vi "FGV Ausgaenge erzwingen.vi"(8 "Aktionen":T1) -> (0 "Aktionen":T1)   [LabVIEW 2020, in "cRIO Ueberwachung.lvlib"]
uses:
  cRIO Ueberwachung.lvlib
  FGV Ausgaenge erzwingen Aktionen.ctl
  Stoerungen/Stoerungen Messgeraet/Aktionen Kommunikation Stoerung.ctl
  Stoerungen/Stoerungen.lvlib
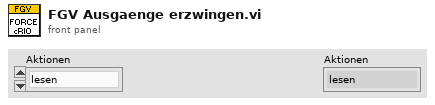
[diagram p1: front panel]
types:
  T1 = typedef "cRIO Ueberwachung.lvlib/FGV Ausgaenge erzwingen Aktionen.ctl" = enum16{"lesen", "starten", "erzwingen", "beenden"}
  T2 = typedef "Stoerungen.lvlib/Aktionen Kommunikation Stoerung.ctl" = enum16{"lesen", "init", "FT-IR Komm", "FT-IR Betriebsart", "FT-IR Hintergrund", "cRIO Komm", "PNS Komm", "Dichtheitstest", "Life Bit", "FTIR Komm AK", "PMA Komm", "FID Komm", "PMA Cal", "FID Ch4 Cal", "FID THC Cal", "Cal Timeout", "VFS 1 Komm", "VFS 2 Komm", "VFS 3 Komm", "VFS 4 Komm", "TRE 08 Komm", "CG-Test vorzeitig", "CG-Test Span 1", "CG-Test Span 2", "CG-Test Span 3", "CG-Test Messgas", "CG-Test löschen", "Test", "Amium AK", "AK Recept konfig", "AK Name konfig", "AK EKFG konfig"}
  T3 = typedef "Stoerungen.lvlib/Stoerungen Messgeraete.ctl" = cluster{"FT-IR Komm":bool, "FT-IR Betriebsart":bool, "FT-IR Hintergrundscan":bool, "Dichtheitstest":bool, "cRIO Komm":bool, "PNS Komm":bool, "Life Bit":bool, "FT-IR AK Komm":bool, "PMA Komm":bool, "FID Komm":bool, "PMA Cal":bool, "FID CH4 Cal":bool, "FID THC Cal":bool, "Cal Timeout":bool, "VFS 1 Komm":bool, "VFS 2 Komm":bool, "VFS 3 Komm":bool, "VFS 4 Komm":bool, "TRE 08 Komm":bool, "CG-Test":bool, "CG-Test 1":bool, "CG-Test 2":bool, "CG-Test 3":bool, "Messgas - Eingang":bool, "Amium AK Komm":bool, "AK Rezept nicht konfiguriert ":bool, "AK Name nicht konfiguriert":bool, "AK EKFG nicht konfiguriert":bool}
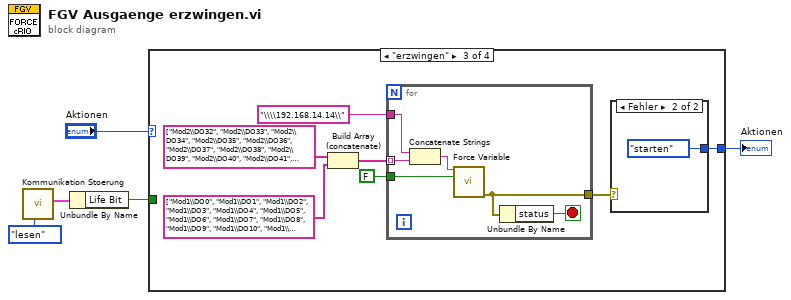
[diagram p0: block diagram]
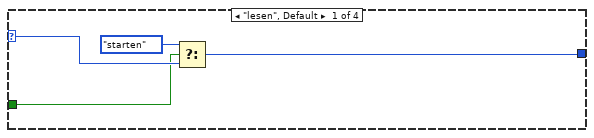
[diagram p2: hidden frame]
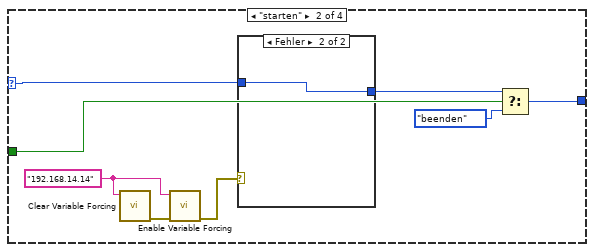
[diagram p3: hidden frame]
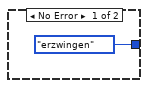
[diagram p4: hidden frame]
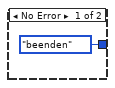
[diagram p5: hidden frame]
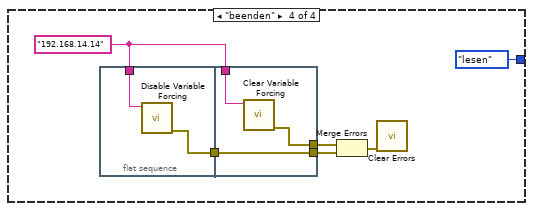
[diagram p6: hidden frame]
diagram:
  n1 = call "Kommunikation Stoerung.vi"("Aktionen"=Aktionen_Kommunikation_Stoerung."lesen") -> ("Störung Messgerät"=w3:T3)  [unwired: 10 in]
  n2 = Unbundle By Name(w3) -> ("Life Bit"=w1:bool)
  n3 = case shown="\"erzwingen\"" "Aktionen" {
    selector: "Aktionen" -> [w9 w12 _ _]
    tunnel: [w7 w10 w24 FGV_Ausgaenge_erzwingen_Aktionen."lesen" ("f")] -> w4
    tunnel: w1 -> [w6 w14 _ _]
    frame "lesen", Default {
      n4 = Select(t=FGV_Ausgaenge_erzwingen_Aktionen."starten", s=w6, f=w9) -> (s? t:f=w7:T1)
    }
    frame "starten" {
      w15 = "192.168.14.14"
      n5 = call <vilib>:"Clear Variable Forcing.vi"("target address (localhost)"=w15) -> ("error out"=w17:errorcluster)  [unwired: 1 in, 7 out]
      n6 = call <vilib>:"Enable Variable Forcing.vi"("error in (no error)"=w17, "target address (localhost)"=w15) -> ("error out"=w16:errorcluster)  [unwired: 7 out]
      n7 = case shown="Fehler" w16 {
        tunnel: [FGV_Ausgaenge_erzwingen_Aktionen."erzwingen" ("Aktionen") w19] -> w11
        tunnel: w12 -> [_ w19]
        frame No Error {
        }
        frame Error {
        }
      }
      n8 = Select(t=w11, s=w14, f=FGV_Ausgaenge_erzwingen_Aktionen."beenden") -> (s? t:f=w10:T1)
    }
    frame "erzwingen" {
      n9 = Build Array (concatenate)(string[] ["Mod2\\DO32", "Mod2\\DO33", "Mod2\\DO34", "Mod2\\DO35", "Mod2\\DO36", "Mod2\\DO37", "Mod2\\DO38", "Mod2\\DO39", "Mod2\\DO40", "Mod2\\DO41", "Mod2\\DO42", "Mod2\\DO43", "Mod2\\DO44", "Mod2\\DO45", "Mod2\\DO46", "Mod2\\DO47", "Mod3\\DO48", "Mod3\\DO49", "Mod3\\DO50", "Mod3\\DO51", "Mod3\\DO52", "Mod3\\DO53", "Mod3\\DO54", "Mod3\\DO55", "Mod3\\DO56", "Mod3\\DO57", "Mod3\\DO58", "Mod3\\DO59", "Mod3\\DO60", "Mod3\\DO61", "Mod3\\DO62", "Mod3\\DO63"], string[] ["Mod1\\DO0", "Mod1\\DO1", "Mod1\\DO2", "Mod1\\DO3", "Mod1\\DO4", "Mod1\\DO5", "Mod1\\DO6", "Mod1\\DO7", "Mod1\\DO8", "Mod1\\DO9", "Mod1\\DO10", "Mod1\\DO11", "Mod1\\DO12", "Mod1\\DO13", "Mod1\\DO14", "Mod1\\DO15", "Mod1\\DO16", "Mod1\\DO17", "Mod1\\DO18", "Mod1\\DO19", "Mod1\\DO20", "Mod1\\DO21", "Mod1\\DO22", "Mod1\\DO23", "Mod1\\DO24", "Mod1\\DO25", "Mod1\\DO26", "Mod1\\DO27", "Mod1\\DO28", "Mod1\\DO29", "Mod1\\DO30", "Mod1\\DO31", "Mod1\\DO32"]) -> (w21:string[])
      n10 = for {
        tunnel: FALSE -> [w34]
        tunnel: w21 -> [w30] mode=indexing
        tunnel: [w33] -> w25
        tunnel: "\\\\192.168.14.14\\" -> [w31]
        stop <- w32 stop-if-true
        n11 = Concatenate Strings(w31, w30) -> (w29:string)
        n12 = call <vilib>:"Force Variable.vi"("variable path (URL)"=w29, "forced value"=w34) -> ("error out"=w33:errorcluster)  [unwired: 1 in, 12 out]
        n13 = Unbundle By Name(w33) -> ("status"=w32:bool)
      }
      n14 = case shown="Fehler" w25 {
        tunnel: [FGV_Ausgaenge_erzwingen_Aktionen."beenden" ("f") FGV_Ausgaenge_erzwingen_Aktionen."starten" ("f")] -> w24
        frame No Error {
        }
        frame Error {
        }
      }
    }
    frame "beenden" {
      w35 = "192.168.14.14"
      n15 = flat-sequence {
        tunnel: [w42] -> w37
        tunnel: w35 -> [w41]
        tunnel: [w45] -> w40
        tunnel: w37 -> [w45]
        tunnel: [w44] -> w36
        tunnel: w35 -> [w43]
        frame #0 {
          n16 = call <vilib>:"Disable Variable Forcing.vi"("target address (localhost)"=w41) -> ("error out"=w42:errorcluster)  [unwired: 1 in, 7 out]
        }
        frame #1 {
          n17 = call <vilib>:"Clear Variable Forcing.vi"("target address (localhost)"=w43) -> ("error out"=w44:errorcluster)  [unwired: 1 in, 7 out]
        }
      }
      n18 = Merge Errors(w36, w40) -> (w39:errorcluster)
      n19 = call <vilib>:"Clear Errors.vi"("error in (no error)"=w39) -> ()  [unwired: 5 in, 2 out]
    }
  }
  "Aktionen" <- w4
